vi "ConvertGoop2ToGoop3_CreateLvClass.vi"(0 "ClassFolder":path, 1 "ProjectItem":refnum<vi>, 5 "ClassName":string, 7 "ViRefsIn":refnum<vi>[](array[refnum]), 9 "ViPathsIn":path[](array[path]), 11 "error in":errorcluster) -> (4 "LvClassCreated":refnum<vi>, 8 "ViRefsOut":refnum<vi>[](array[refnum]), 10 "ViPathsOut":path[](array[path]), 15 "error out":errorcluster)   [LabVIEW 2012]
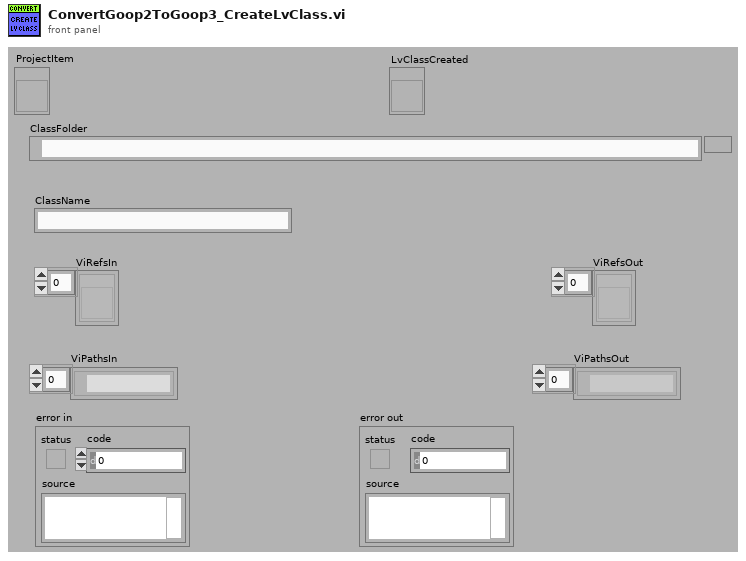
[diagram p1: front panel]
types:
  T1 = enum32{"invalid scope", "public", "private", "protected"}
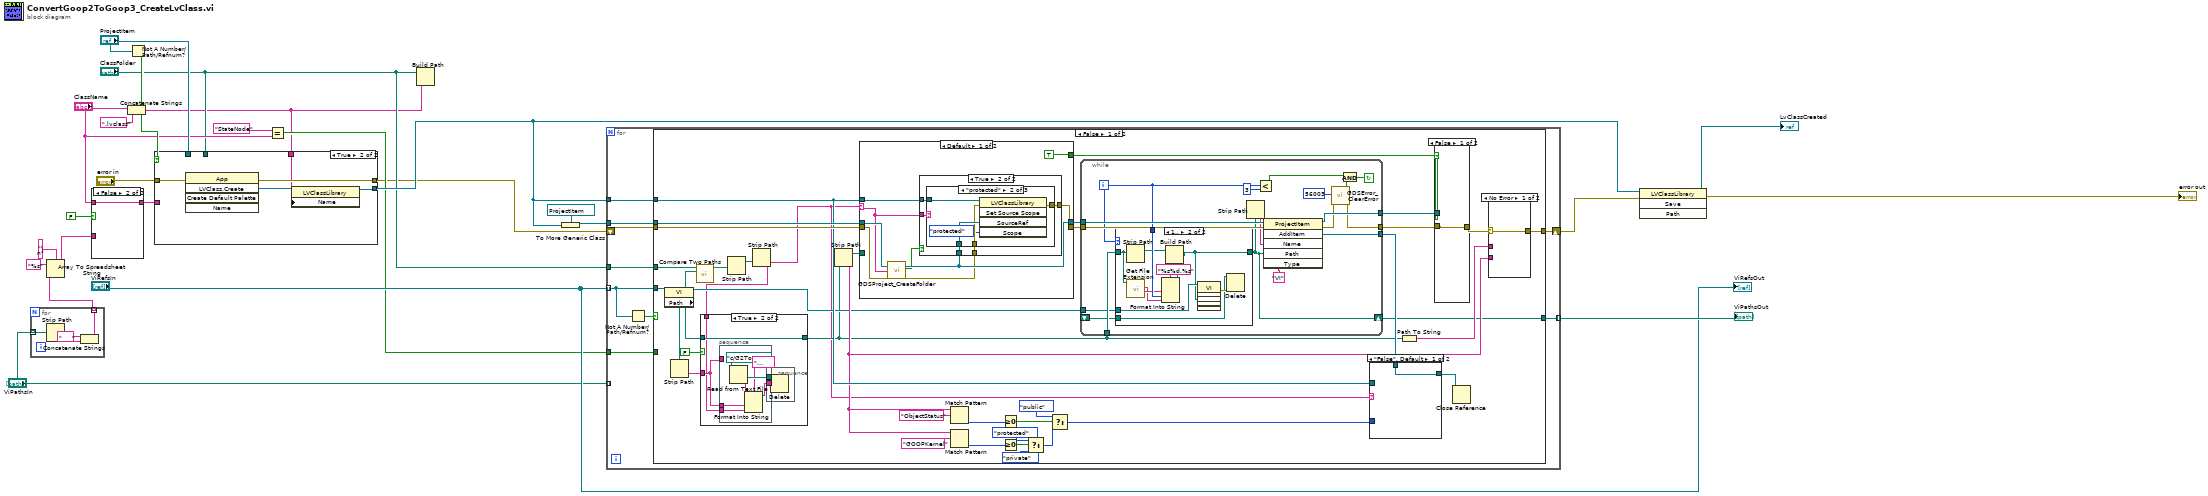
[diagram p0: block diagram]
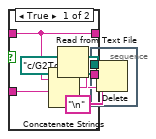
[diagram p2: hidden frame]
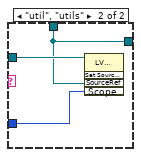
[diagram p6: hidden frame]
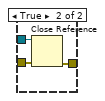
[diagram p7: hidden frame]
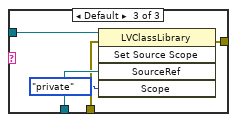
[diagram p10: hidden frame]
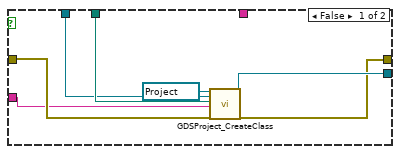
[diagram p13: hidden frame]
diagram:
  n1 = for {
    tunnel: "ViPathsIn" -> [w29] mode=indexing
    tunnel: [w26] -> w11 mode=indexing
    n2 = Strip Path(path=w29) -> (name=w28:string)  [unwired: 1 out]
    n3 = Concatenate Strings("     " ("string"), w28) -> (w26:string)
  }
  n4 = Array To Spreadsheet String(delimiter (Tab)="\n", array=w11, 3:"%s" ("format string")) -> (spreadsheet string=w8:string)
  n5 = case shown="False" FALSE {
    tunnel: "ClassName" -> [w32 w39]
    tunnel: [w32 w39] -> w13
    tunnel: w8 -> [w30 _]
    frame True {
      w35 = path "c:/G2To3.txt" ("file (use dialog)")
      w31 = "\n" ("string")
      n6 = Read from Text File(file (use dialog)=w35) -> (text=w33:string)  [unwired: 3 in, 3 out]
      n7 = Concatenate Strings(w33, w32, w31, w30, w31) -> (w34:string)
      n8 = stacked-sequence {
        tunnel: w34 -> [w38]
        tunnel: w35 -> [w36]
        frame #0 {
          n9 = Delete(path (use dialog)=w36) -> (deleted path=w37:path)  [unwired: 4 in, 2 out]
          n10 = Write to Text File(file (use dialog)=w37, text=w38) -> ()  [unwired: 2 in, 3 out]
        }
      }
    }
    frame False {
    }
  }
  n11 = Concatenate Strings("ClassName", ".lvclass" ("string")) -> (w2:string)
  n12 = Not A Number/Path/Refnum?(number/path/refnum="ProjectItem") -> (NaN/Path/Refnum?=w22:bool)
  n13 = case shown="True" w22 {
    tunnel: "error in" -> [w44 w51]
    tunnel: [w46 w47] -> w18
    tunnel: [w45 w50] -> w1
    tunnel: "ProjectItem" -> [w41 _]
    tunnel: w13 -> [w43 _]
    tunnel: "ClassFolder" -> [w42 _]
    tunnel: w2 -> [_ w48]
    frame False {
      n14 = call <resource>:"GDSProject_CreateClass.vi"("Project Refnum In"=refnum<vi> refnum, "Project Item To Create Class Below(Use MyComputer if not wired)"=w41, "ClassFolder"=w42, "ClassName"=w43, "error in (no error)"=w44) -> ("Class Refnum Out"=w46:refnum<vi>, "error out"=w45:errorcluster)  [unwired: 11 in, 2 out]
    }
    frame True {
      n15 = invoke class="App" method="LVClass.Create"(error in=w51) -> (error out=w50:errorcluster, "LVClass.Create"=w49:refnum<vi>)  [unwired: 4 in, 3 out]
      n16 = property class="LVClassLibrary"(reference=w49, "Name"=w48) -> (reference out=w47:refnum<vi>)  [unwired: 1 in, 1 out]
    }
  }
  n17 = Equal?(x="StateNode" ("Type"), y="ClassName") -> (x = y?=w5:bool)
  n18 = Build Path(base path="ClassFolder", name or relative path=w2) -> ()  [unwired: 1 out]
  n19 = To More Generic Class(target class=refnum<vi> refnum ("AddItem"), reference=w18) -> (generic class reference=w19:refnum<vi>)
  n20 = for {
    tunnel: w19 -> [w60]
    shift-right: [w56] -> w16
    shift-left: w1 -> [w59]
    tunnel: w18 -> [w58]
    tunnel: "ViRefsIn" -> [w54] mode=indexing
    tunnel: "ClassFolder" -> [w57]
    tunnel: "ViPathsIn" -> [_] mode=indexing
    tunnel: [w55] -> w15 mode=indexing
    tunnel: w5 -> [w52]
    n21 = Not A Number/Path/Refnum?(number/path/refnum=w54) -> (NaN/Path/Refnum?=w53:bool)
    n22 = case shown="False" w53 {
      tunnel: w60 -> [w95 _]
      tunnel: w59 -> [w93 w178]
      tunnel: w58 -> [w90 _]
      tunnel: w57 -> [w74 _]
      tunnel: [w72 w178] -> w56
      tunnel: [w68 _] -> w55
      tunnel: w54 -> [w67 _]
      tunnel: w52 -> [_ _]
      frame False {
        n23 = property class="VI"(reference=w67) -> (reference out=w66:refnum<vi>, "Path"=w64:path)  [unwired: 1 in, 1 out]
        n24 = Strip Path(path=w64) -> (name=w63:string)  [unwired: 1 out]
        n25 = call <vilib>:"Compare Two Paths.vi"("Path 2"=w64, "Path 1"=w74) -> ("Relative Path from 1 to 2"=w76:path)  [unwired: 6 in, 3 out]
        n26 = Strip Path(path=w76) -> (stripped path=w75:path)  [unwired: 1 out]
        n27 = Strip Path(path=w75) -> (name=w62:string)  [unwired: 1 out]
        n28 = case shown="True" FALSE {
          tunnel: w64 -> [w98 w101]
          tunnel: [w98 w101] -> w65
          tunnel: w63 -> [_ w100]
          tunnel: w62 -> [_ w99]
          frame False {
          }
          frame True {
            n29 = stacked-sequence {
              tunnel: w100 -> [_]
              tunnel: w100 -> [w103]
              tunnel: w99 -> [w102]
              frame #0 {
                w107 = path "c:/G2To3.txt" ("file (use dialog)")
                n30 = Read from Text File(file (use dialog)=w107) -> (text=w104:string)  [unwired: 3 in, 3 out]
                n31 = Format Into String(format string="       %s(%s)\n", initial string=w104, w103, w102) -> (resulting string=w106:string)  [unwired: 1 in, 1 out]
                n32 = stacked-sequence {
                  tunnel: w106 -> [w110]
                  tunnel: w107 -> [w108]
                  frame #0 {
                    n33 = Delete(path (use dialog)=w108) -> (deleted path=w109:path)  [unwired: 4 in, 2 out]
                    n34 = Write to Text File(file (use dialog)=w109, text=w110) -> ()  [unwired: 2 in, 3 out]
                  }
                }
              }
            }
          }
        }
        n35 = Strip Path(path=w65) -> (stripped path=w96:path, name=w71:string)
        n36 = case shown="Default" w62 {
          selector: w62 -> [w152 _]
          tunnel: w95 -> [w158 w177]
          tunnel: [w155 w177] -> w94
          tunnel: w93 -> [w157 w176]
          tunnel: [w153 w176] -> w97
          tunnel: w96 -> [_ _]
          tunnel: w90 -> [w156 _]
          tunnel: [TRUE _] -> w91
          frame Default {
            n37 = call <resource>:"GDSProject_CreateFolder.vi"("Project Item To Create Folder Below(Use MyComputer if not wired)"=w158, "FolderName"=w152, "error in (no error)"=w157) -> ("ItemOut"=w155:refnum<vi>, "FolderCreated"=w150:bool, "error out"=w154:errorcluster)  [unwired: 13 in, 1 out]
            n38 = case shown="True" w150 {
              tunnel: w156 -> [_ w164]
              tunnel: w155 -> [_ w163]
              tunnel: w154 -> [w159 w162]
              tunnel: [w159 w161] -> w153
              tunnel: w152 -> [_ w160]
              frame False {
              }
              frame True {
                n39 = case shown="\"protected\"" w160 {
                  tunnel: w164 -> [_ w170 w175]
                  tunnel: w163 -> [_ w169 w174]
                  tunnel: w162 -> [w165 w168 w173]
                  tunnel: [w165 w167 w172] -> w161
                  frame "Public", "util", "utils" {
                  }
                  frame "protected" {
                    n40 = invoke class="LVClassLibrary" method="Set Source Scope"(reference=w170, error in=w168, "SourceRef"=w169, "Scope"=T1."protected" ("scope")) -> (error out=w167:errorcluster)  [unwired: 1 in, 4 out]
                  }
                  frame Default {
                    n41 = invoke class="LVClassLibrary" method="Set Source Scope"(reference=w175, error in=w173, "SourceRef"=w174, "Scope"=T1."private" ("scope")) -> (error out=w172:errorcluster)  [unwired: 1 in, 4 out]
                  }
                }
              }
            }
          }
          frame "" {
          }
        }
        n42 = Match Pattern(string=w71, regular expression="ObjectStatus") -> (offset past match=w88:i32)  [unwired: 1 in, 3 out]
        n43 = Match Pattern(string=w71, regular expression="GOOPKernel") -> (offset past match=w83:i32)  [unwired: 1 in, 3 out]
        n44 = Greater Or Equal To 0?(x=w88) -> (x >= 0?=w87:bool)
        n45 = Greater Or Equal To 0?(x=w83) -> (x >= 0?=w82:bool)
        n46 = Select(t=T1."protected" ("scope"), s=w82, f=T1."private" ("scope")) -> (s? t:f=w81:T1)
        n47 = Select(t=T1."public" ("scope"), s=w87, f=w81) -> (s? t:f=w85:T1)
        n48 = while {
          tunnel: w97 -> [w128]
          tunnel: w94 -> [w127]
          tunnel: [w125] -> w92
          tunnel: [w124] -> w78
          tunnel: [w121] -> w69
          tunnel: w65 -> [w116]
          tunnel: w66 -> [w114]
          shift-right: [w112] -> w68
          shift-left: _ -> [w113]
          i -> [w115]
          stop <- w117 continue-if-true
          n49 = case shown="1.." w115 {
            tunnel: w116 -> [w129 w140]
            tunnel: [w129 w132] -> w112
            tunnel: w115 -> [_ w138]
            tunnel: w114 -> [_ w133]
            tunnel: w113 -> [_ w130]
            frame Default {
            }
            frame 1.. {
              n50 = Strip Path(path=w140) -> (stripped path=w135:path)  [unwired: 1 out]
              n51 = call <vilib>:"Get File Extension.vi"("file"=w140) -> ("filename without extension"=w137:string, "lowercase file extension"=w136:string)  [unwired: 7 in, 2 out]
              n52 = Format Into String(format string="%s%d.%s", w137, w138, w136) -> (resulting string=w134:string)  [unwired: 2 in, 1 out]
              n53 = Build Path(base path=w135, name or relative path=w134) -> (appended path=w132:path)
              n54 = invoke class="VI" method="Save.Instrument"(reference=w133, "Path to saved file"=w132) -> (error out=w131:errorcluster)  [unwired: 4 in, 5 out]
              n55 = Delete(path (use dialog)=w130, error in=w131) -> ()  [unwired: 3 in, 3 out]
            }
          }
          n56 = Strip Path(path=w112) -> (name=w111:string)  [unwired: 1 out]
          n57 = Less?(x=w115, y=3) -> (x < y?=w119:bool)
          n58 = invoke class="ProjectItem" method="AddItem"(reference=w127, error in=w128, "Name"=w111, "Path"=w112, "Type"="VI") -> (reference out=w125:refnum<vi>, error out=w122:errorcluster, "AddItem"=w124:refnum<vi>)  [unwired: 1 in, 3 out]
          n59 = call <resource>:"GDSError_ClearError.vi"("code"=56003, "error in (no error)"=w122) -> ("Cleared?"=w118:bool, "error out"=w121:errorcluster)  [unwired: 16 in]
          n60 = And(x=w119, y=w118) -> (x .and. y?=w117:bool)
        }
        n61 = case shown="\"False\", Default" w62 {
          tunnel: w78 -> [w142 w143]
          tunnel: w90 -> [_ w145]
          tunnel: w85 -> [_ w144]
          tunnel: [w142 w143] -> w77
          frame "False", Default {
          }
          frame "util", "utils" {
            n62 = invoke class="LVClassLibrary" method="Set Source Scope"(reference=w145, "SourceRef"=w143, "Scope"=w144) -> ()  [unwired: 2 in, 5 out]
          }
        }
        n63 = Path To String(path=w65) -> (string=w70:string)
        n64 = case shown="False" w91 {
          tunnel: w69 -> [w146 w149]
          tunnel: [w146 w148] -> w73
          tunnel: w92 -> [_ w147]
          frame False {
          }
          frame True {
            n65 = Close Reference(reference=w147, error in (no error)=w149) -> (error out=w148:errorcluster)
          }
        }
        n66 = Close Reference(reference=w77) -> ()  [unwired: 1 in, 1 out]
        n67 = case shown="No Error" w73 {
          selector: w73 -> [w141 _]
          tunnel: [w141 _] -> w72
          tunnel: w71 -> [_ _]
          tunnel: w70 -> [_ _]
          frame No Error {
          }
          frame Error {
          }
        }
      }
      frame True {
      }
    }
  }
  "ViPathsOut" <- w15
  n68 = invoke class="LVClassLibrary" method="Save"(reference=w18, error in=w16) -> (reference out=→"LvClassCreated":refnum<vi>, error out=→"error out":errorcluster)  [unwired: 2 in, 2 out]
  "ViRefsOut" <- "ViRefsIn"
